vi "Set Cell Value (Timestamp).vi"(6 "Value":timestamp format="%<%x %.3X>T", 8 "error in":errorcluster, 9 "Cell Address":string, 10 "Worksheet":refnum<k24>, 11 "SpreadsheetDoc in":refnum<k24>) -> (0 "error out":errorcluster, 2 "Worksheet out":refnum<k24>, 3 "SpreadsheetDoc out":refnum<k24>)   [LabVIEW 2019, in "Open Xml.lvlib"]
uses:
  Open Xml.lvlib
  D:/git/Open-Xml-LabVIEW/Source/DocumentFormat.OpenXml.dll
  DocumentFormat.OpenXml.dll
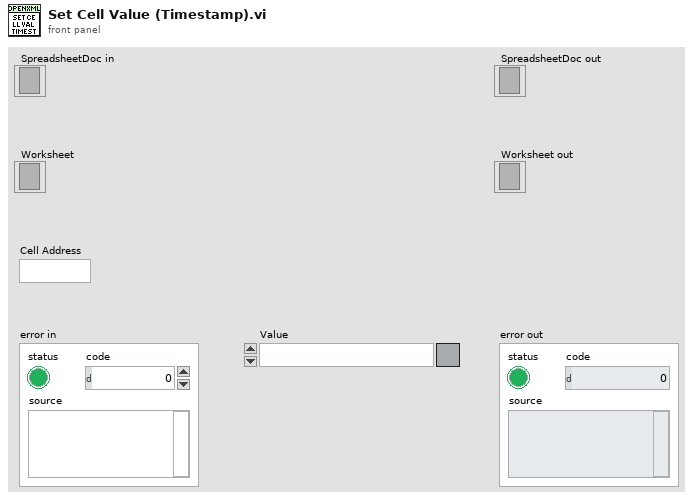
[diagram p1: front panel]
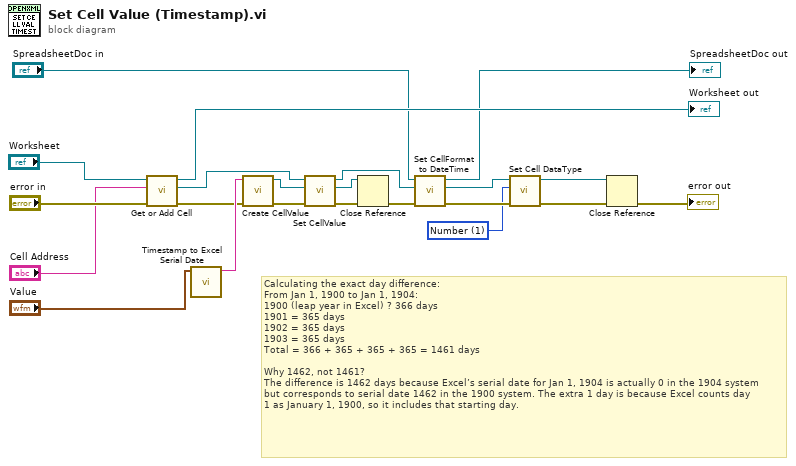
[diagram p0: block diagram]
diagram:
  w7 = 1 items=["Boolean", "Number", "Error", "SharedString", "String", "InlineString", "Date"] ("Datatype")
  # "Calculating the exact day difference:\nFrom Jan 1, 1900 to Jan 1, 1904:\n1900 (leap year in Excel) ? 366 days\n1901 = 365 days\n1902 = 365 days\n1903 = 365 days\nTotal = 366 + 365 + 365 + 365 = 1461 days\n\nWhy 1462, not 1461?\nThe difference is 1462 days because Excel’s serial date for Jan 1, 1904 is actually 0 in the 1904 system\nbut corresponds to serial date 1462 in the 1900 system. The extra 1 day is because Excel counts day\n1 as January 1, 1900, so it includes that starting day."
  n1 = call "Get or Add Cell.vi"("error in"="error in", "Cell Address"="Cell Address", "Worksheet in"="Worksheet") -> ("error out"=w9:errorcluster, "Cell"=w10:refnum<k24>, "Worksheet out"=→"Worksheet out":refnum<k24>)  [unwired: 6 in]
  n2 = call "Timestamp to Excel Serial Date.vi"("Timestamp"="Value") -> ("Excel Serial Date"=w12:string)  [unwired: 10 in]
  n3 = call "Create CellValue.vi"("error in"=w9, "Text"=w12) -> ("error out"=w4:errorcluster, "CellValue out"=w8:refnum<k24>)  [unwired: 8 in]
  n4 = call "Set CellValue.vi"("error in"=w4, "CellValue in"=w8, "Cell in"=w10) -> ("error out"=w6:errorcluster, "CellValue out"=w22:refnum<k24>, "Cell out"=w14:refnum<k24>)  [unwired: 6 in]
  n5 = Close Reference(reference=w22, error in (no error)=w6) -> (error out=w21:errorcluster)
  n6 = call "Set CellFormat to DateTime.vi"("error in"=w21, "Cell in"=w14, "SpreadsheetDoc in"="SpreadsheetDoc in") -> ("error out"=w13:errorcluster, "Cell out"=w15:refnum<k24>, "SpreadsheetDoc out"=→"SpreadsheetDoc out":refnum<k24>)  [unwired: 6 in]
  n7 = call "Set Cell DataType.vi"("error in"=w13, "Datatype"=w7, "Cell in"=w15) -> ("error out"=w5:errorcluster, "Cell out"=w19:refnum<k24>)  [unwired: 7 in]
  n8 = Close Reference(reference=w19, error in (no error)=w5) -> (error out=→"error out":errorcluster)
